vi "UMLEditor closeDiagram.vi"(5 "error in (no error)":errorcluster, 6 "localVariablesIn":T2 {"ObjectHotspots"."HotSpot"."y" format="%.2f"; "ObjectHotspots"."HotSpot"."x" format="%.2f"; "NodesBounds"."height" format="%.2f"; "NodesBounds"."width" format="%.2f"; "NodesBounds"."y" format="%.2f"; "NodesBounds"."x" format="%.2f"; "offset"."y" format="%.2f"; "offset"."x" format="%.2f"; "gridSize" format="%.2f"; "dragStartBounds"."height" format="%.2f"; "dragStartBounds"."width" format="%.2f"; "dragStartBounds"."y" format="%.2f"; "dragStartBounds"."x" format="%.2f"; "dragStartPoint"."y" format="%.2f"; "dragStartPoint"."x" format="%.2f"; "rubberBandStart"."y" format="%.2f"; "rubberBandStart"."x" format="%.2f"; "lastMousePoint"."y" format="%.2f"; "lastMousePoint"."x" format="%.2f"; "zoom" format="%.2f"}) -> (12 "localVariablesOut":T2 {"ObjectHotspots"."HotSpot"."y" format="%.2f"; "ObjectHotspots"."HotSpot"."x" format="%.2f"; "NodesBounds"."height" format="%.2f"; "NodesBounds"."width" format="%.2f"; "NodesBounds"."y" format="%.2f"; "NodesBounds"."x" format="%.2f"; "offset"."y" format="%.2f"; "offset"."x" format="%.2f"; "gridSize" format="%.2f"; "dragStartBounds"."height" format="%.2f"; "dragStartBounds"."width" format="%.2f"; "dragStartBounds"."y" format="%.2f"; "dragStartBounds"."x" format="%.2f"; "dragStartPoint"."y" format="%.2f"; "dragStartPoint"."x" format="%.2f"; "rubberBandStart"."y" format="%.2f"; "rubberBandStart"."x" format="%.2f"; "lastMousePoint"."y" format="%.2f"; "lastMousePoint"."x" format="%.2f"; "zoom" format="%.2f"}, 15 "lastDiagramClosed":bool, 16 "diagramType":T1, 19 "error out":errorcluster)   [LabVIEW 2014]
doc: "Gets current diagram values"
uses:
  <resource>/Framework/Providers/Open_GDS/UML/UMLEditor/UMLEditor LocalVariablesType.ctl
  <resource>/Framework/Providers/Open_GDS/UML/Graphics_class/Graphics.lvclass
  <resource>/Framework/Providers/Open_GDS/UML/Grid_class/Grid.lvclass
  <resource>/Framework/Providers/Open_GDS/UML/AbstractEdge_class/AbstractEdge.lvclass
  <resource>/Framework/Providers/Open_GDS/UML/AbstractNode_class/AbstractNode.lvclass
  <resource>/Framework/Providers/Open_GDS/UML/UMLEditor/UMLEditor statesType.ctl
  <resource>/Framework/Providers/Open_GDS/UML/UMLEditor/UMLEditor tooltype.ctl
  <resource>/Framework/Providers/Open_GDS/UML/UMLEditor/UMLEditor_DiagramInfo.ctl
  <resource>/Framework/Providers/Open_GDS/UML/Graph_class/Graph.lvclass
  <resource>/Framework/Providers/Open_GDS/UML/General/Point/Point Point2D.ctl
  <resource>/Framework/Providers/Open_GDS/UML/General/Rectangle/Rectangle Rectangle2D.ctl
  <resource>/Framework/Providers/Open_GDS/UML/UMLEditor/UMLEditor ExportType.ctl
  <resource>/Framework/Providers/Open_GDS/UML/UMLEditor/UMLEditor FlattenCommandType.ctl
  <resource>/Framework/Providers/Open_GDS/UML/UMLEditor/UMLEditor ExecuteCommandType.ctl
  <resource>/Framework/Providers/Open_GDS/UML/ContextHelp/ContextHelp_EventType.ctl
  <resource>/Framework/Providers/Open_GDS/UML/UMLEditor/UMLEditor_HotSpotData.ctl
  <resource>/Framework/Providers/Open_GDS/UML/UMLEditor/UMLEditor_HotSpotType.ctl
  <resource>/Framework/Providers/Open_GDS/UML/UmlEditor_class/EventData.ctl
  <resource>/Framework/Providers/Open_GDS/UML/UMLEditor/UMLEditor_DiagramType.ctl
  <resource>/Framework/Providers/Open_GDS/UML/UmlEditor_class/UmlEditor.lvclass
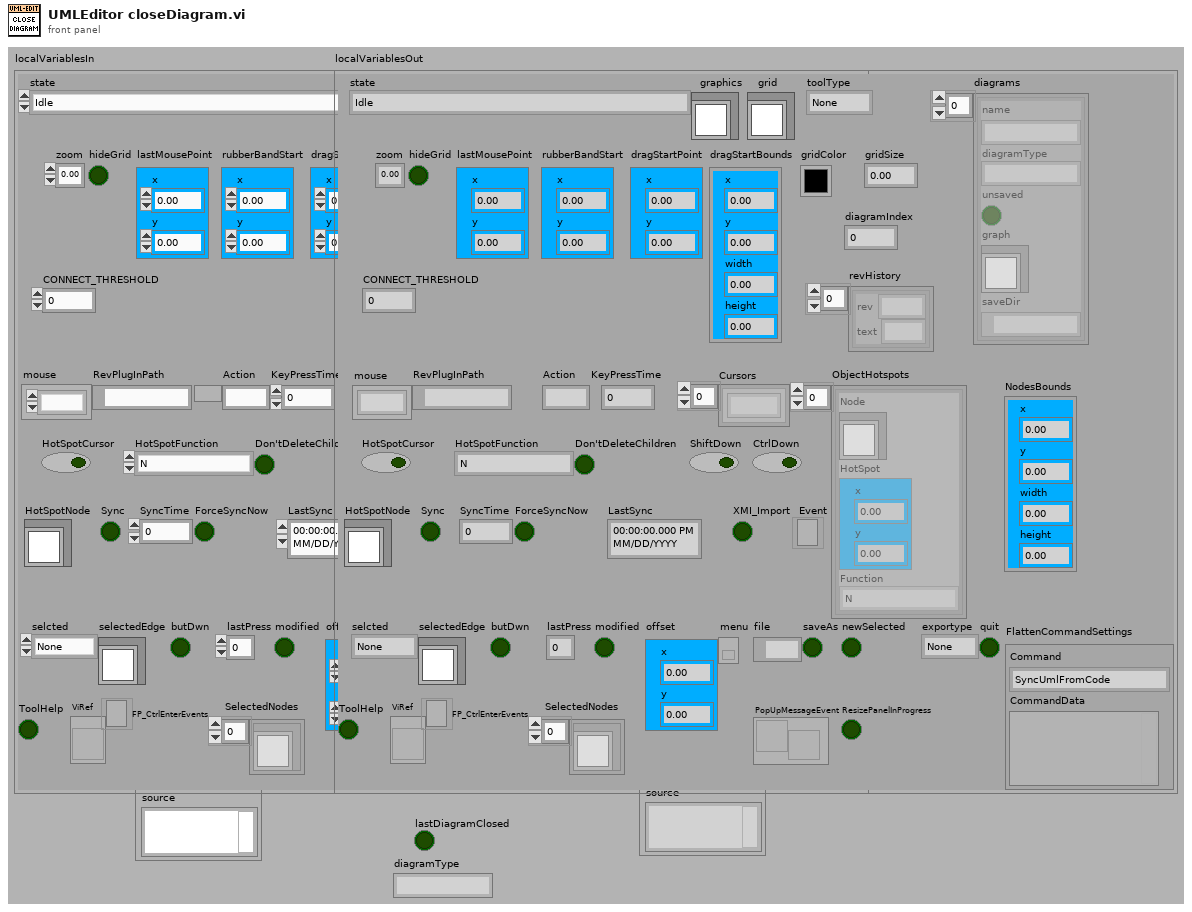
[diagram p1: front panel]
types:
  T1 = typedef "UMLEditor_DiagramType.ctl" = string
  T2 = typedef "UMLEditor LocalVariablesType.ctl" = cluster{"state":T3, "graphics":refnum<class "Graphics.lvclass">, "grid":refnum<class "Grid.lvclass">, "toolType":T4, "diagramIndex":i32, "diagrams":T5[], "zoom":dbl, "hideGrid":bool, "lastMousePoint":T6, "rubberBandStart":T6, "dragStartPoint":T6, "dragStartBounds":T7, "gridColor":u32, "gridSize":dbl, "CONNECT_THRESHOLD":i32, "selcted":T4, "selectedEdge":refnum<class "AbstractEdge.lvclass">, "butDwn":bool, "lastPress":u32, "modified":bool, "offset":T6, "menu":refnum<k9>, "file":path, "saveAs":bool, "newSelected":bool, "exportype":T8, "quit":bool, "revHistory":cluster{"rev":string, "text":string}[], "FlattenCommandSettings":T9, "PopUpMessageEvent":T11, "ResizePanelInProgress":bool, "NodesBounds":T7, "ToolHelp":bool, "ViRef":refnum<vi>, "FP_CtrlEnterEvents":refnum<event-registration>, "SelectedNodes":refnum<class "AbstractNode.lvclass">[], "mouse":refnum<k1>, "RevPlugInPath":path, "Action":string, "KeyPressTime":u32, "Cursors":refnum<k1>[], "ObjectHotspots":T12[], "HotSpotCursor":bool, "HotSpotFunction":T13, "Don'tDeleteChildren":bool, "ShiftDown":bool, "CtrlDown":bool, "HotSpotNode":refnum<class "AbstractNode.lvclass">, "Sync":bool, "SyncTime":u32, "ForceSyncNow":bool, "LastSync":timestamp, "XMI_Import":bool, "Event":refnum<event-registration>}
  T3 = typedef "UMLEditor statesType.ctl" = enum16{"Idle", "CheckLicense", "revHistory", "Init", "Init2", "EditSelected", "RemoveSelected", "PaintComponent", "ChangeZoom", "ChangeGridSize", "Open", "Close", "Save", "ExportPicture", "Export", "Repaint", "Error", "Exit", "QUIT", "CreateScript", "ExecuteScript", "ClassReversedEngineering", "PlugInReverseEngineering", "StateReversedEngineering", "AutoPlace", "ExecuteCommand", "OpenClass", "SyncAll", "StraightenAssociation", "Copy", "Paste", "AddNodeFromProjectTree", "AddNodeFromProjectTree+SyncAll", "PanAndRepaint", "Init3", "CopyPaste", "ApplyDesignPattern", "AnalyseViInStateDiagram", "AutoSync"}
  T4 = typedef "UMLEditor tooltype.ctl" = enum16{"None", "Node", "Edge"}
  T5 = typedef "UMLEditor_DiagramInfo.ctl" = cluster{"name":string, "diagramType":string, "unsaved":bool, "graph":refnum<class "Graph.lvclass">, "saveDir":path}
  T6 = typedef "Point Point2D.ctl" = cluster{"x":dbl, "y":dbl}
  T7 = typedef "Rectangle Rectangle2D.ctl" = cluster{"x":dbl, "y":dbl, "width":dbl, "height":dbl}
  T8 = typedef "UMLEditor ExportType.ctl" = enum16{"None", "Printer", "png", "jpg", "roseUML"}
  T9 = typedef "UMLEditor FlattenCommandType.ctl" = cluster{"Command":T10, "CommandData":variant}
  T10 = typedef "UMLEditor ExecuteCommandType.ctl" = enum16{"SyncUmlFromCode", "SyncCodeFromUML", "OpenClass", "OpenFile", "CreateClass", "CreateVI", "OpenClassAttribute", "LocateInProject"}
  T11 = typedef "ContextHelp_EventType.ctl" = refnum<user-event>
  T12 = typedef "UMLEditor_HotSpotData.ctl" = cluster{"Node":refnum<class "AbstractNode.lvclass">, "HotSpot":T6, "Function":T13}
  T13 = typedef "UMLEditor_HotSpotType.ctl" = enum16{"N", "NE", "E", "SE", "S", "SW", "W", "NW", "Expand", "Collaps"}
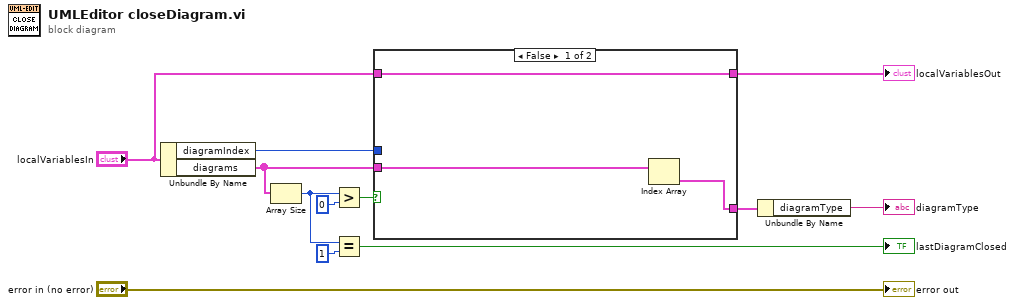
[diagram p0: block diagram]
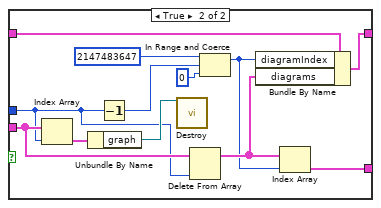
[diagram p2: hidden frame]
diagram:
  n1 = Unbundle By Name("localVariablesIn") -> ("diagramIndex"=w3:i32, "diagrams"=w4:T5[])
  n2 = Array Size(array=w4) -> (size(s)=w2:i32)
  n3 = Greater?(x=w2, y=0) -> (0:w5:bool)
  n4 = Equal?(x=w2, y=1) -> (x = y?=→"lastDiagramClosed":bool)
  n5 = case shown="False" w5 {
    tunnel: "localVariablesIn" -> [w15 w27]
    tunnel: [w15 w26] -> w10
    tunnel: w4 -> [w14 w21]
    tunnel: w3 -> [_ w20]
    tunnel: [w13 w16] -> w8
    frame False {
      n6 = Index Array(array=w14) -> (element=w13:T5)  [unwired: 1 in]
    }
    frame True {
      n7 = Index Array(array=w21, index=w20) -> (element=w19:T5)
      n8 = Unbundle By Name(w19) -> ("graph"=w22:refnum<class "Graph.lvclass">)
      n9 = Decrement(x=w20) -> (x-1=w25:i32)
      n10 = call-dynamic "Destroy.vi"("reference"=w22) -> ()  [unwired: 18 in, 1 out]
      n11 = Delete From Array(array=w21, index=w20) -> (array with subset deleted=w18:T5[])  [unwired: 1 in, 1 out]
      n12 = In Range and Coerce(upper limit=2147483647, x=w25, lower limit=0) -> (coerced(x)=w17:i32)  [unwired: 1 out]
      n13 = Bundle By Name(cluster=w27, "diagramIndex"=w17, "diagrams"=w18) -> (w26:T2)
      n14 = Index Array(array=w18, index=w17) -> (element=w16:T5)
    }
  }
  "localVariablesOut" <- w10
  n15 = Unbundle By Name(w8) -> ("diagramType"=→"diagramType":string)
  "error out" <- "error in (no error)"
